vi "9229通道配置全局.vi"() -> ()   [LabVIEW 2013]
panel:
  out "9229通道配置全局":bool[](array[boolean])
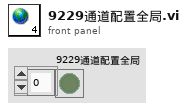
[diagram p1: front panel]
diagram:
